vi "Send with Error Check.vi"(8 "error in (no error)":errorcluster, 10 "Command":string, 11 "7976A in":refnum<class "7976A.lvclass">) -> (0 "error out":errorcluster, 3 "7976A out":refnum<class "7976A.lvclass">)   [LabVIEW 2019, in "7976A.lvlib" / "7976A.lvclass"]
uses:
  Library/7976A.lvclass
  Library/7976A.lvclass/7976A.ctl
  <instrlib>/Agilent N7976A/Agilent N7976A.lvlib
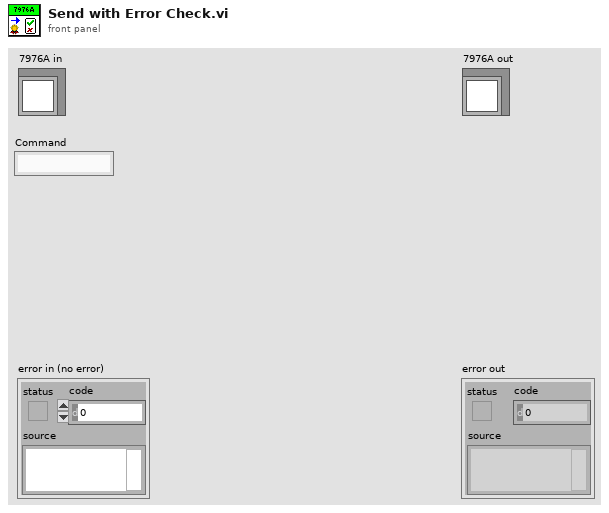
[diagram p1: front panel]
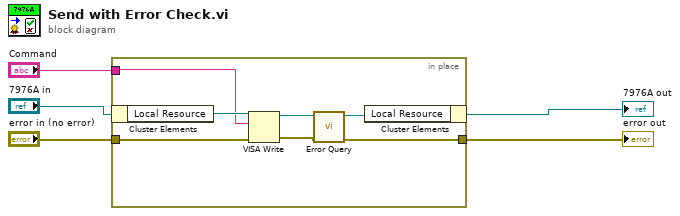
[diagram p0: block diagram]
diagram:
  n1 = in-place {
    in-place-border: [w8] -> w3
    in-place-border: "error in (no error)" -> [w7]
    in-place-border: "Command" -> [w6]
    n2 = in-place-cluster #1("7976A in") -> ("Local Resource"=w10:refnum<visa-resource-name>)
    n3 = VISA Write(VISA resource name=w10, write buffer=w6, error in (no error)=w7) -> (VISA resource name out=w11:refnum<visa-resource-name>, error out=w12:errorcluster)  [unwired: 1 out]
    n4 = call <instrlib>:"Error Query.vi"("error in (no error)"=w12, "VISA resource name"=w11) -> ("error out"=w8:errorcluster, "VISA resource name out"=w9:refnum<visa-resource-name>)  [unwired: 6 in, 2 out]
    n5 = in-place-cluster #1("Local Resource"=w9) -> (→"7976A out":refnum<class "7976A.lvclass">)
  }
  "error out" <- w3
